vi "FABR-Dispose Of Data.vi"(0 "Path":path) -> (8 "Deleted":bool)   [LabVIEW 2020]
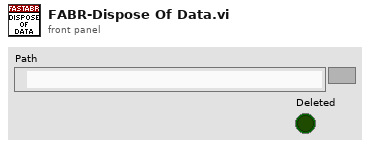
[diagram p1: front panel]
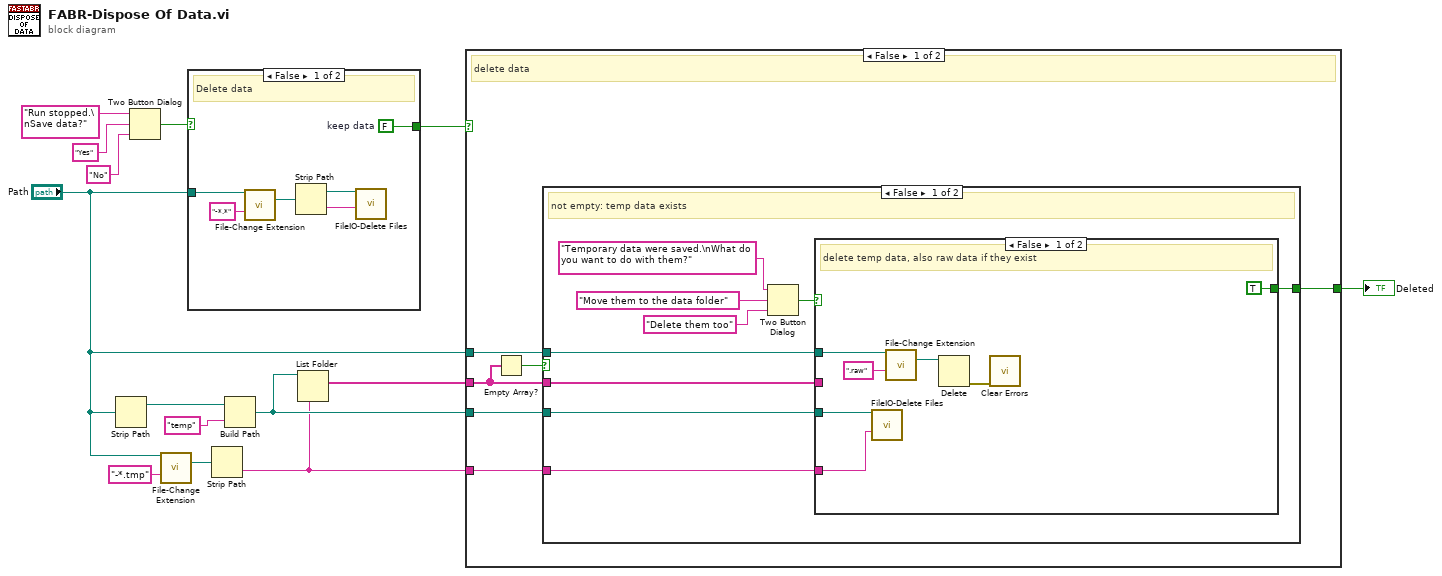
[diagram p0: block diagram]
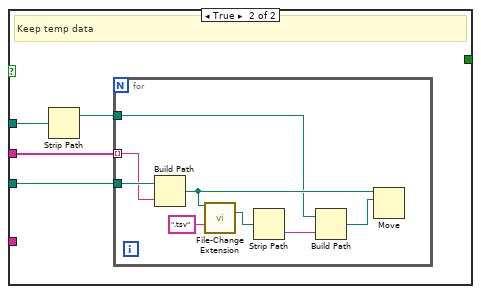
[diagram p2: hidden frame]
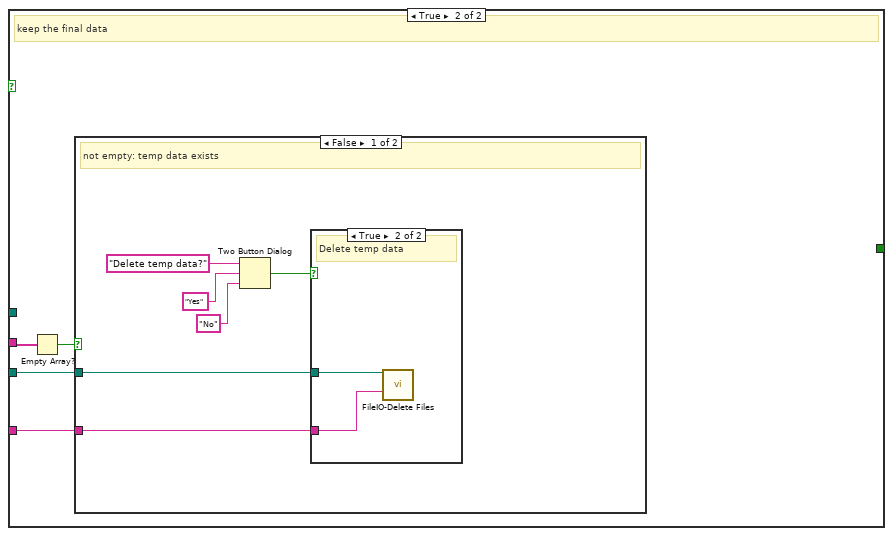
[diagram p4: hidden frame]
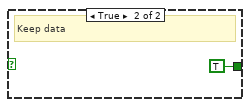
[diagram p7: hidden frame]
diagram:
  n1 = Strip Path(path="Path") -> (stripped path=w10:path)  [unwired: 1 out]
  n2 = Two Button Dialog(message="Run stopped.\nSave data?", 1:"No" ("F button name (\"Cancel\")"), 2:"Yes" ("T button name (\"OK\")")) -> (T button?=w14:bool)
  n3 = call "File-Change Extension.vi"("Path"="Path", "new extension"="-*.tmp") -> ("new path"=w7:path)  [unwired: 12 in, 1 out]
  n4 = case shown="False" w14 {
    tunnel: "Path" -> [w16 _]
    tunnel: [w15 TRUE] -> w6
    frame False {
      w15 = FALSE  # keep data
      # "Delete data"
      n5 = call "File-Change Extension.vi"("Path"=w16, "new extension"="-*.*") -> ("new path"=w17:path)  [unwired: 12 in, 1 out]
      n6 = Strip Path(path=w17) -> (stripped path=w20:path, name=w18:string)
      n7 = call "FileIO-Delete Files.vi"("Folder"=w20, "Pattern"=w18) -> ()  [unwired: 13 in, 1 out]
    }
    frame True {
      # "Keep data"
    }
  }
  n8 = Strip Path(path=w7) -> (name=w4:string)  [unwired: 1 out]
  n9 = Build Path(base path=w10, name or relative path="temp") -> (appended path=w5:path)
  n10 = List Folder(path=w5, pattern=w4) -> (filenames=w2:string[])  [unwired: 2 in, 3 out]
  n11 = case shown="False" w6 {
    tunnel: w5 -> [w27 w59]
    tunnel: w4 -> [w26 w58]
    tunnel: "Path" -> [w25 _]
    tunnel: w2 -> [w23 w56]
    tunnel: [w22 _] -> w1
    frame False {
      # "delete data"
      n12 = Empty Array?(array=w23) -> (empty?=w24:bool)
      n13 = case shown="False" w24 {
        tunnel: w27 -> [w32 _]
        tunnel: w26 -> [w31 _]
        tunnel: w25 -> [w30 _]
        tunnel: w23 -> [w29 _]
        tunnel: [w28 _] -> w22
        frame False {
          # "not empty: temp data exists"
          n14 = Two Button Dialog(message="Temporary data were saved.\nWhat do you want to do with them?", 1:"Delete them too" ("T button name (\"OK\")"), 2:"Move them to the data folder" ("F button name (\"Cancel\")")) -> (T button?=w33:bool)
          n15 = case shown="False" w33 {
            tunnel: w32 -> [w43 w44]
            tunnel: w31 -> [w42 _]
            tunnel: w30 -> [w38 w46]
            tunnel: w29 -> [_ w47]
            tunnel: [TRUE _] -> w28
            frame False {
              # "delete temp data, also raw data if they exist"
              n16 = call "FileIO-Delete Files.vi"("Folder"=w43, "Pattern"=w42) -> ()  [unwired: 13 in, 1 out]
              n17 = call "File-Change Extension.vi"("Path"=w38, "new extension"=".raw") -> ("new path"=w41:path)  [unwired: 12 in, 1 out]
              n18 = Delete(path (use dialog)=w41) -> (error out=w39:errorcluster)  [unwired: 4 in, 2 out]
              n19 = call <vilib>:"Clear Errors.vi"("error in (no error)"=w39) -> ()  [unwired: 5 in, 2 out]
            }
            frame True {
              # "Keep temp data"
              n20 = Strip Path(path=w46) -> (stripped path=w45:path)  [unwired: 1 out]
              n21 = for {
                tunnel: w47 -> [w54] mode=indexing
                tunnel: w45 -> [w50]
                tunnel: w44 -> [w55]
                n22 = Build Path(base path=w55, name or relative path=w54) -> (appended path=w53:path)
                n23 = call "File-Change Extension.vi"("Path"=w53, "new extension"=".tsv") -> ("new path"=w51:path)  [unwired: 12 in, 1 out]
                n24 = Strip Path(path=w51) -> (name=w49:string)  [unwired: 1 out]
                n25 = Build Path(base path=w50, name or relative path=w49) -> (appended path=w48:path)
                n26 = Move(source path=w53, 10:w48) -> ()  [unwired: 3 in, 3 out]
              }
            }
          }
        }
        frame True {
        }
      }
    }
    frame True {
      # "keep the final data"
      n27 = Empty Array?(array=w56) -> (empty?=w57:bool)
      n28 = case shown="False" w57 {
        tunnel: w59 -> [w61 _]
        tunnel: w58 -> [w60 _]
        frame False {
          # "not empty: temp data exists"
          n29 = Two Button Dialog(message="Delete temp data?", 1:"No" ("F button name (\"Cancel\")"), 2:"Yes" ("T button name (\"OK\")")) -> (T button?=w62:bool)
          n30 = case shown="True" w62 {
            tunnel: w61 -> [_ w67]
            tunnel: w60 -> [_ w66]
            frame False {
            }
            frame True {
              # "Delete temp data"
              n31 = call "FileIO-Delete Files.vi"("Folder"=w67, "Pattern"=w66) -> ()  [unwired: 13 in, 1 out]
            }
          }
        }
        frame True {
          # "no temp data to dispose"
        }
      }
    }
  }
  "Deleted" <- w1
